vi "Estructura de Datos.vi"() -> ()   [LabVIEW 2020]
panel:
  in  "Meter":dbl(knob) scale=0.0..10.0
  out "Knob":dbl(knob) scale=0.0..10.0
  # "3 ESTRUCTURAS DE DATOS\n- Control\n- Indicador\n- Constante"
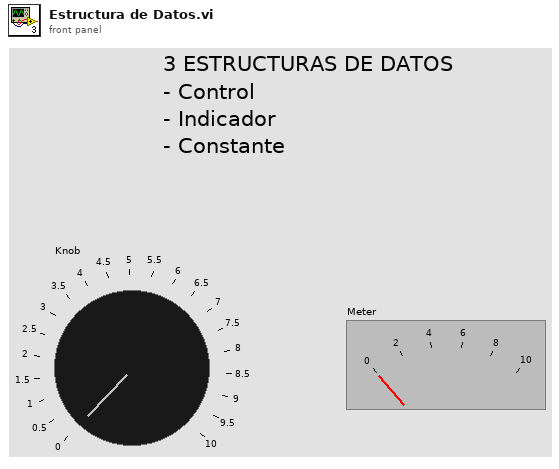
[diagram p1: front panel]
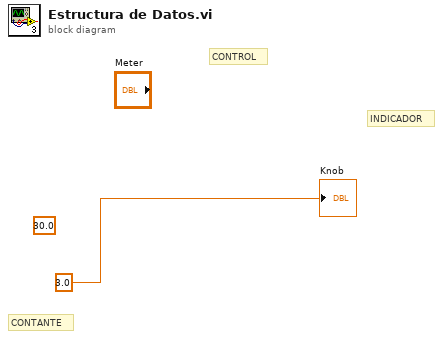
[diagram p0: block diagram]
diagram:
  (unwired) 30.0
  # "CONTANTE"
  # "INDICADOR"
  # "CONTROL"
  "Knob" <- 3.0
